vi "In Acceptable Range.vi"(9 "Variable":dbl, 10 "Setpoint":dbl, 11 "Acceptable Range":dbl) -> (3 "Boolean":bool)   [LabVIEW 2018]
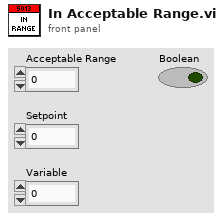
[diagram p1: front panel]
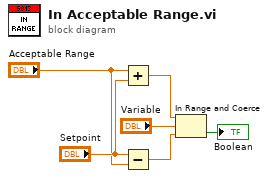
[diagram p0: block diagram]
diagram:
  n1 = Add(x="Acceptable Range", y="Setpoint") -> (x+y=w2:dbl)
  n2 = Subtract(x="Setpoint", y="Acceptable Range") -> (x-y=w1:dbl)
  n3 = In Range and Coerce(upper limit=w2, x="Variable", lower limit=w1) -> (In Range?=→"Boolean":bool)  [unwired: 1 out]
